vi "getWavFileWaveform.vi"(8 "error in (no error)":errorcluster, 11 "path to .WAV file":path) -> (0 "error out":errorcluster, 1 "sample rate (S/s)":dbl, 2 "total number of samples/ch":u32, 3 "audio waveform array":waveform(dbl)[](array[waveform]), 4 "right channel out":waveform(dbl), 6 "left channel out":waveform(dbl))   [LabVIEW 2020]
doc: "This VI returns a waveform array containing data from a WAV file. Currently only designed for stereo WAV files."
uses:
  <vilib>/sound2/lvsound2.llb/Sound File Read Open.vi
  <vilib>/sound2/lvsound2.llb/Sound File Info (refnum).vi
  <vilib>/sound2/lvsound2.llb/Sound File Read (DBL).vi
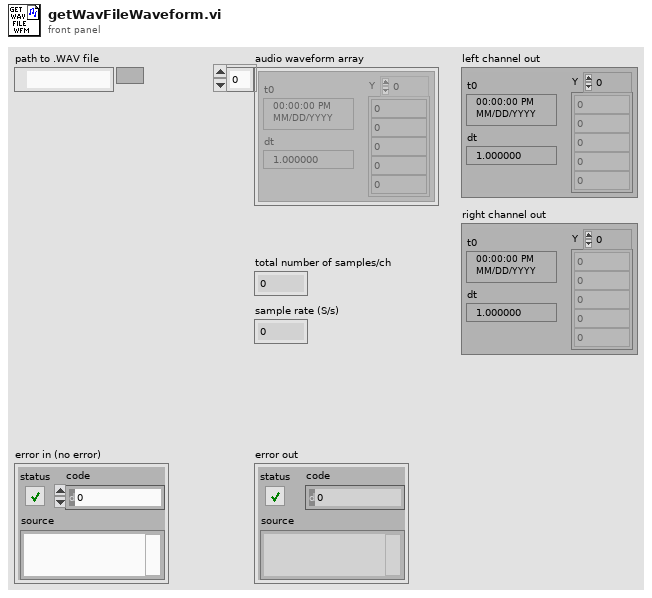
[diagram p1: front panel]
types:
  T1 = typedef "Sound File Refnum.ctl" = refnum<file>
  T2 = typedef "Sound Data Format.ctl" = cluster{"sample rate (S/s)":dbl, "number of channels":i32, "bits per sample":i32}
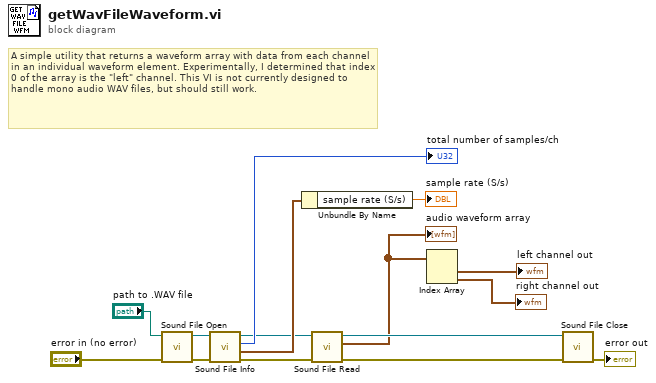
[diagram p0: block diagram]
diagram:
  # "A simple utility that returns a waveform array with data from each channel in an individual waveform element. Experimentally, I determined that index 0 of the array is the \"left\" channel. This VI is not currently designed to handle mono audio WAV files, but should still work."
  n1 = call-poly <vilib>:"Sound File Open.vi"("error in (no error)"="error in (no error)", "path"="path to .WAV file") -> ("error out"=w4:errorcluster, "sound file refnum"=w7:T1)  [unwired: 8 in]
  n2 = call-poly <vilib>:"Sound File Info.vi"("error in (no error)"=w4, "sound file refnum"=w7) -> ("error out"=w5:errorcluster, "sound format"=w11:T2, "total number of samples/ch"=→"total number of samples/ch":u32, "sound file refnum out"=w8:T1)  [unwired: 6 in]
  n3 = Unbundle By Name(w11) -> ("sample rate (S/s)"=→"sample rate (S/s)":dbl)
  n4 = call-poly <vilib>:"Sound File Read.vi"("error in (no error)"=w5, "sound file refnum"=w8) -> ("error out"=w6:errorcluster, "data"=w3:waveform(dbl)[], "sound file refnum out"=w9:T1)  [unwired: 5 in, 2 out]
  "audio waveform array" <- w3
  n5 = Index Array(array=w3) -> (element #1=→"left channel out":waveform(dbl), element #2=→"right channel out":waveform(dbl))  [unwired: 2 in]
  n6 = call <vilib>:"Sound File Close.vi"("error in (no error)"=w6, "sound file refnum"=w9) -> ("error out"=→"error out":errorcluster)  [unwired: 9 in]
